vi "MainGlassCockpitWii.vi"() -> ()   [LabVIEW 2017]
uses:
  Sub_VIs/IMU_Functions/IMU_Data_Cluster.ctl
  Sub_VIs/Instruments/SlipIndicator.ctl
panel:
  out "Design":string
  out "Firmware Revision":string
  out "I2C Error Count":u16
  out "Cycle Time":u16
  out "Read Sensors":bool
  out "GPS-Fix":bool
  in  "EXIT":bool
  in  "ViewSelect":T1(tab)
  out "Boolesch 3":bool
  out "Boolesch 2":bool
  out "MultiWii Data Cluster OUT":T2 {"Altitude abs [m]" format="%.2f"; "Baro T [°C]" format="%.1f"; "Baro P [mbara]" format="%.1f"; "GPS_coord[LON]" format="%#_9f"; "GPS_coord[LAT]" format="%#_9f"; "Altitude [m]" format="%.2f"}
  out "No. of recorded Data":i32
  in  "Ident":bool
  in  "Status":bool
  in  "ACC_Calib.":bool
  in  "Mag_Calib.":bool
  in  "ReadSensorData":bool
  in  "RecordGPS-Data":bool
  in  "RecordFC-Data":bool
  out "COM ok":bool
  in  "COM Port":refnum<visa-resource-name>="COM7"
  in  "Difference Local/UTC [h]":i32=1
  out "GPS":string
  in  "GPS/Baro_Alt":bool
  in  "ScaleUnit(F=m; T=feet)":bool
  out "AltitudeIndicator":picture
  out "AltitudeDigital":dbl
  in  "GPS/Mag":bool
  in  "GPS/Baro_Vario":bool
  out "VerticalSpeedIndicator":picture
  out "VerticalSpeedDigital":dbl format="%.1f"
  out "HeadingDigital":dbl format="%.1f"
  out "TurnBankPlaneIndicator":picture caption="Neue Grafik"
  out "TurnBankStdRate":bool
  in  "ScaleUnit(F=km/h; T=knots)":bool
  out "SpeedIndicator":picture
  out "Local":string
  out "UTC":string
  out "ArtificialHorizon":picture
  out "SlipIndicator":T3 scale=-10.0..10.0
  out "Compass":picture
  # "Set the right COM port first before\nyou run the application !"
  # "on my laptop:\nCOM3-> SE v2.0\nCOM7-> AIOP v2.0"
  # "D - CF2811"
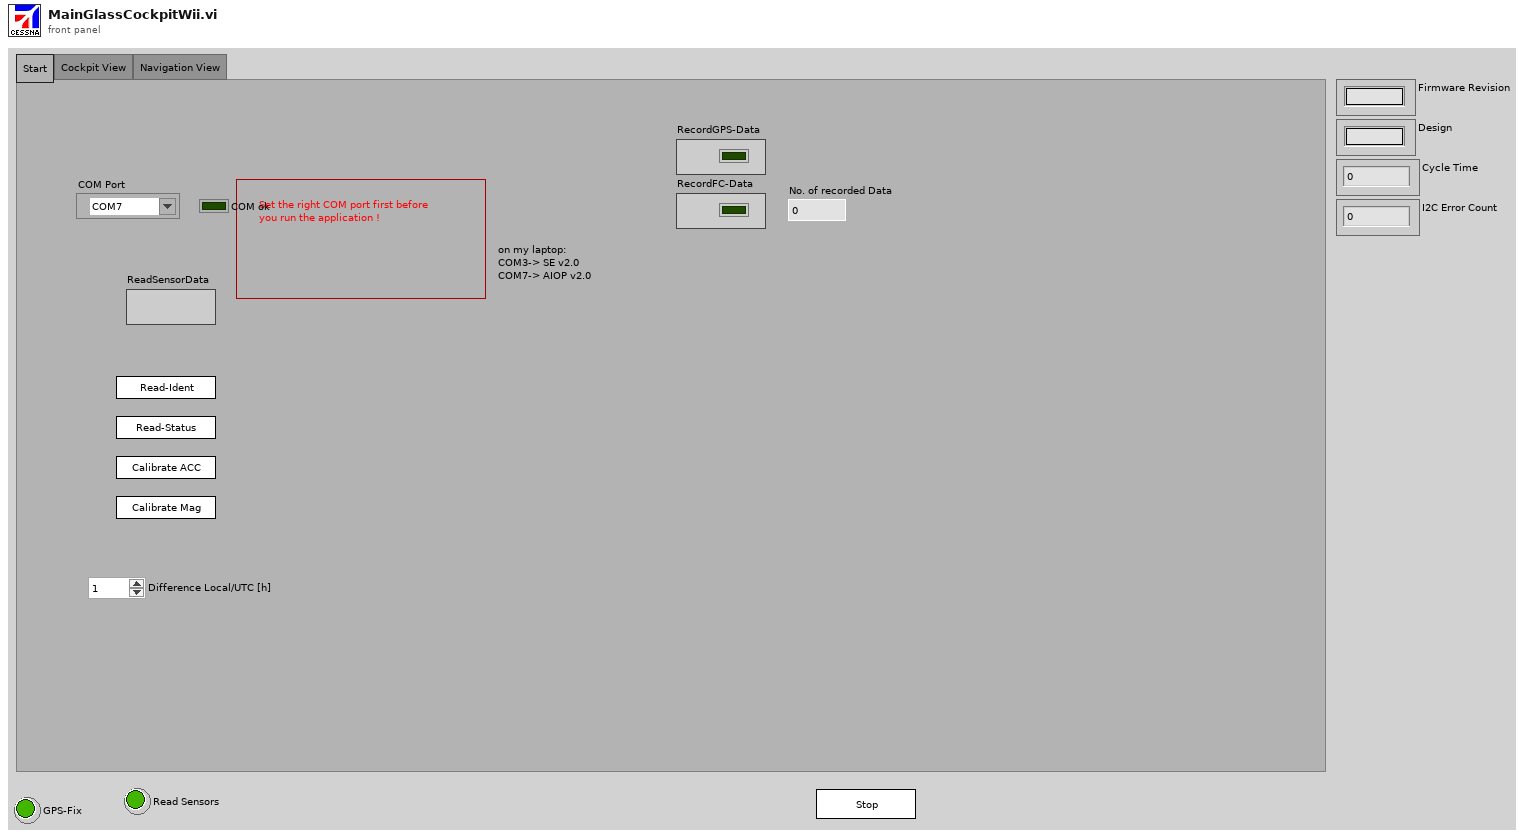
[diagram p1: front panel]
types:
  T1 = enum32{"Start", "Cockpit View", "Navigation View"}
  T2 = typedef "IMU_Data_Cluster.ctl" = cluster{"Firmware Revision":string, "Multitype Name":string, "Cycle Time":u16, "I²C Error Count":u16, "ACC present":bool, "Baro present":bool, "Mag Present":bool, "GPS present":bool, "Sonar present":bool, "Acc X axis (Roll)":dbl, "Acc Y axis (Pitch)":dbl, "Acc Z axis (Yaw)":dbl, "Gyro X axis (Roll)":dbl, "Gyro Y axis (Pitch)":dbl, "Gyro Z axis (Yaw)":dbl, "Mag X axis (Roll)":dbl, "Mag Y axis (Pitch)":dbl, "Mag Z axis (Yaw)":dbl, "X angle (Roll)":dbl, "Y angle (Pitch)":dbl, "Heading [°]":dbl, "Altitude [m]":dbl, "Vario":dbl, "GPS_Fix":u8, "GPS_NumSat":u8, "GPS_coord[LAT]":dbl, "GPS_coord[LON]":dbl, "GPS_Altitude":dbl, "GPS_Speed over Ground":dbl, "GPS_Ground Course":dbl, "Baro P [mbara]":dbl, "Baro T [°C]":dbl, "Altitude abs [m]":dbl}
  T3 = typedef "SlipIndicator.ctl" = dbl
  T4 = enum8{"Enabled", "Disabled", "Disabled and Grayed Out"}
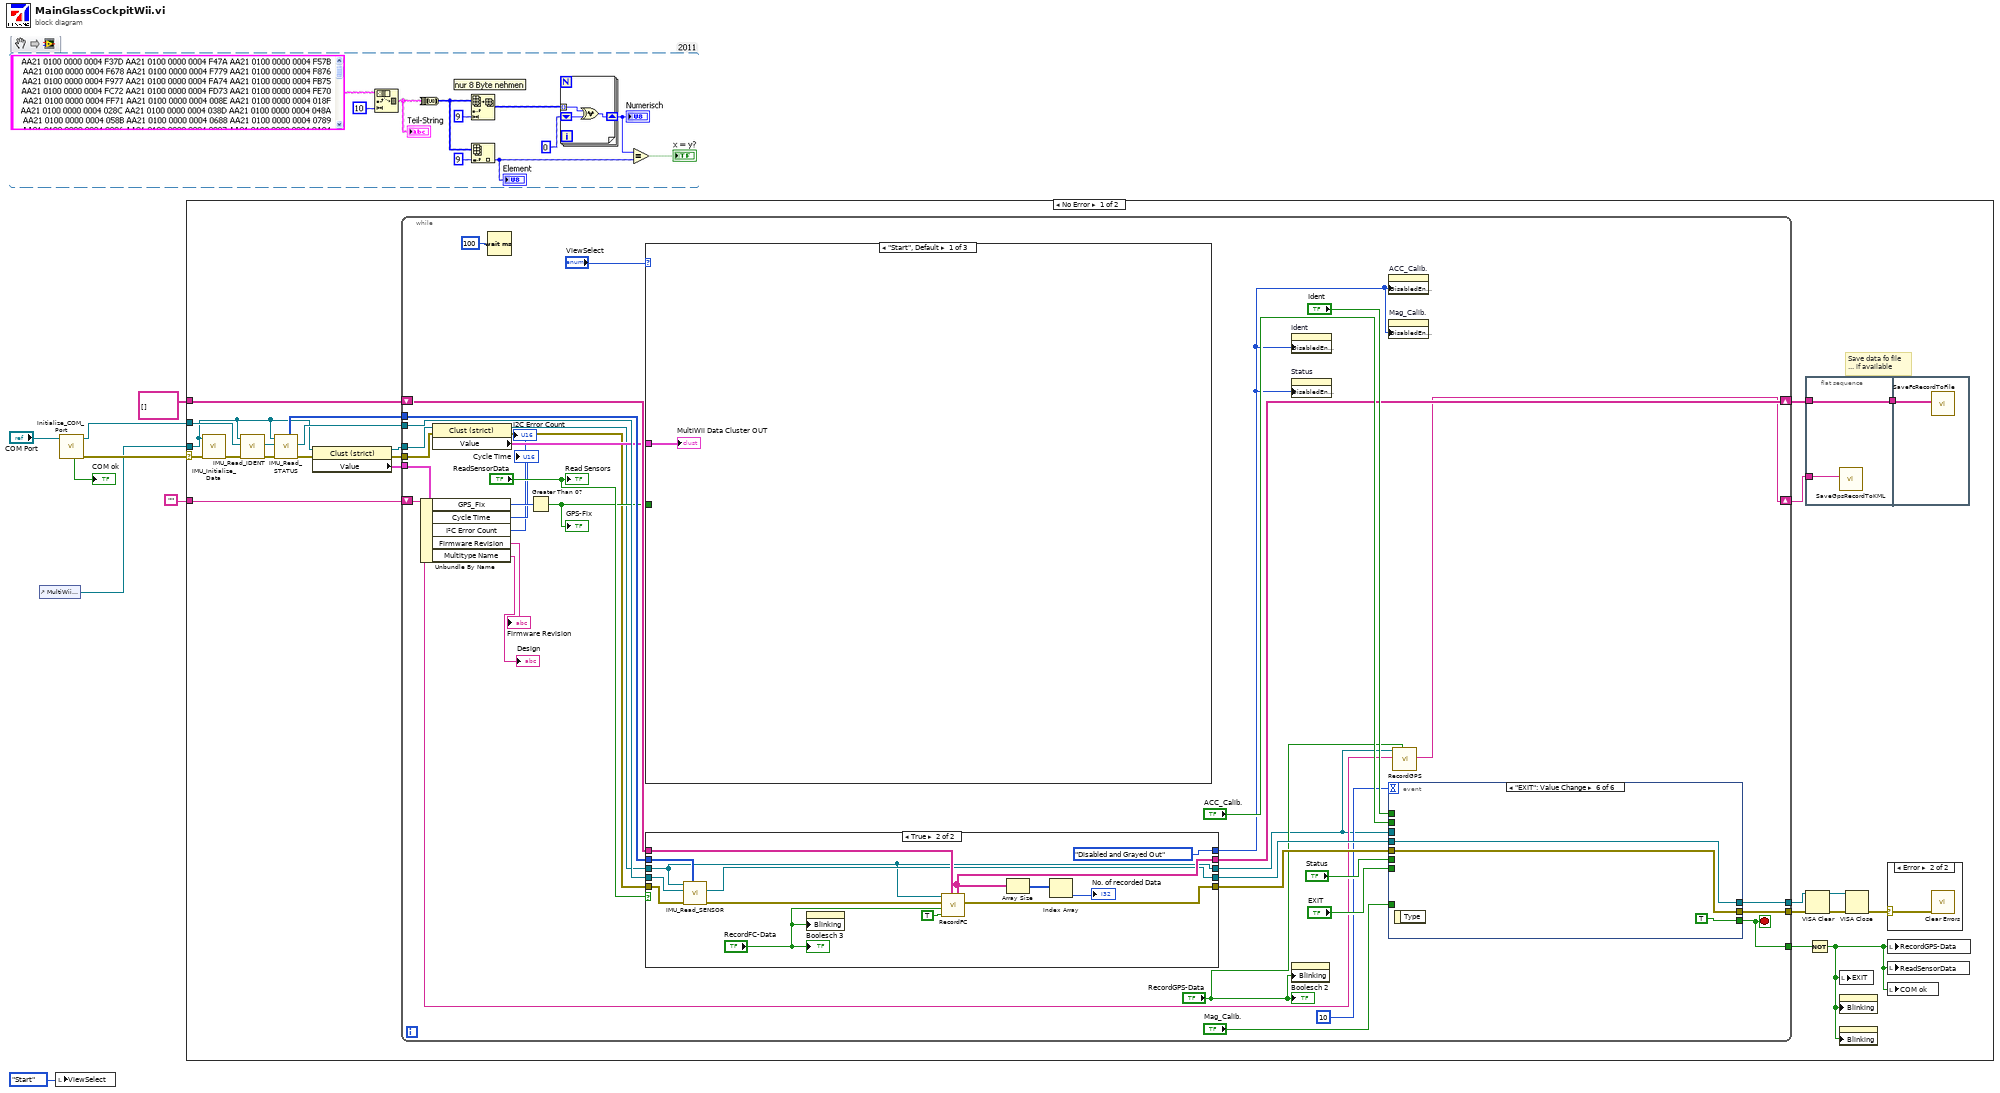
[diagram p0: block diagram]
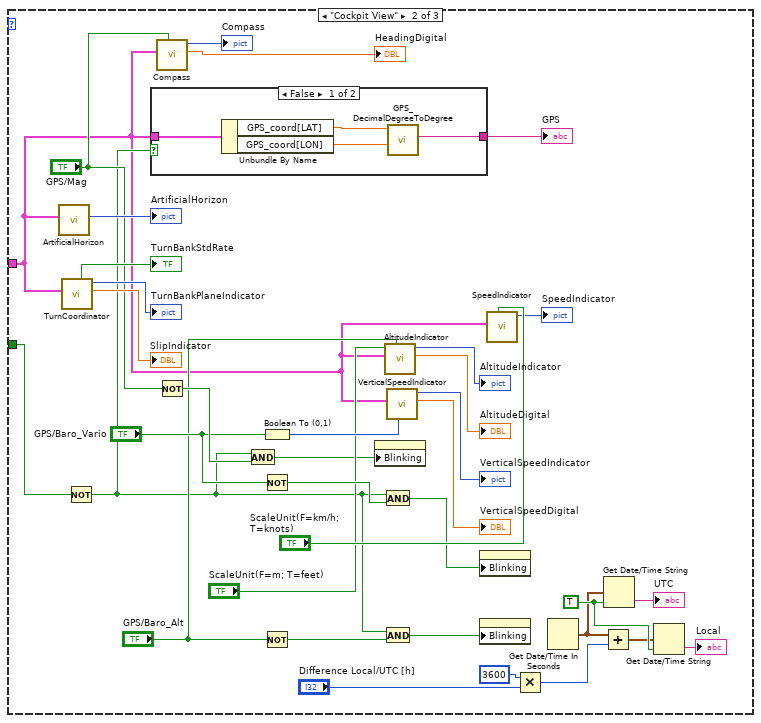
[diagram p3: hidden frame]
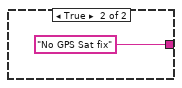
[diagram p4: hidden frame]
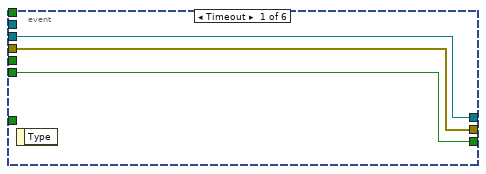
[diagram p6: hidden frame]
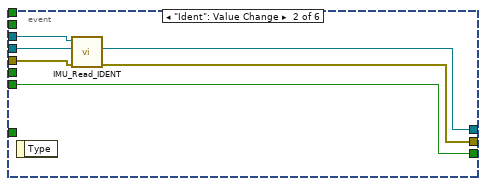
[diagram p7: hidden frame]
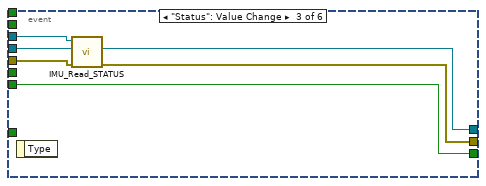
[diagram p8: hidden frame]
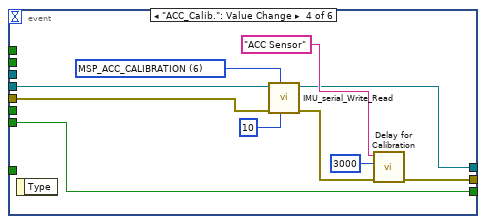
[diagram p9: hidden frame]
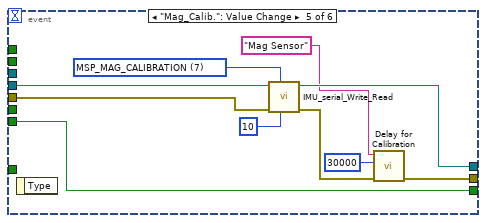
[diagram p10: hidden frame]
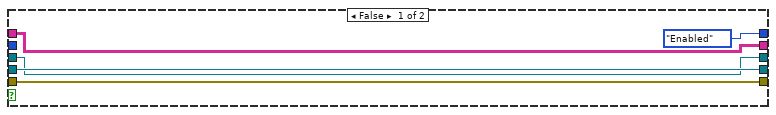
[diagram p11: hidden frame]
diagram:
  n1 = control-ref of="MultiWii Data Cluster OUT"() -> (w1:refnum<vi>)
  n2 = local write "ViewSelect"(T1."Start" ("ViewSelect")) -> ()
  n3 = call "Initialize_COM_Port.vi"("VISA resource name IN"="COM Port") -> ("error out 2"=w8:errorcluster, "VISA resource name OUT"=w7:refnum<visa-resource-name>, "COM ok"=→"COM ok":bool)  [unwired: 8 in]
  n4 = case shown="No Error" w8 {
    selector: w8 -> [w32 _]
    tunnel: w7 -> [w16 _]
    tunnel: "" -> [w22 _]
    tunnel: string[][] [] -> [w21 _]
    tunnel: w1 -> [w13 _]
    frame No Error {
      # "Save data fo file\n... if available"
      n5 = call "IMU_Initialize_Data.vi"("error in (no error)"=w32, "MultiWii Data Cluster"=w13) -> ("error out"=w31:errorcluster)  [unwired: 9 in]
      n6 = call "IMU_Read_IDENT.vi"("error in (no error)"=w31, "VISA resource name IN"=w16, "MultiWii Data Cluster 2"=w13) -> ("error out"=w30:errorcluster, "VISA resource name OUT"=w15:refnum<visa-resource-name>)  [unwired: 7 in]
      n7 = call "IMU_Read_STATUS.vi"("error in (no error)"=w30, "VISA resource name IN"=w15, "MultiWii Data Cluster 2"=w13) -> ("error out"=w12:errorcluster, "VISA resource name OUT"=w14:refnum<visa-resource-name>, "Sensors Present"=w23:u16[])  [unwired: 6 in]
      n8 = property class="Clust (strict)"(reference=w13, error in=w12) -> (reference out=w10:refnum<vi>, error out=w11:errorcluster, "Value"=w9:T2)
      n9 = while {
        tunnel: w14 -> [w71]
        tunnel: w11 -> [w42]
        tunnel: [w62] -> w25
        tunnel: [w64] -> w26
        tunnel: [w60] -> w29
        tunnel: w23 -> [w59]
        shift-right: [w52] -> w17
        shift-left: w22 -> [w53]
        shift-right: [w56] -> w18
        shift-left: w21 -> [w57]
        tunnel: w10 -> [w46]
        tunnel: w9 -> [w45]
        stop <- w60 stop-if-true
        n10 = Unbundle By Name(w45) -> ("GPS_Fix"=w49:u8, "Cycle Time"=→"Cycle Time":u16, "I²C Error Count"=→"I2C Error Count":u16, "Firmware Revision"=→"Firmware Revision":string, "Multitype Name"=→"Design":string)
        n11 = property class="Clust (strict)"(reference=w46, error in=w42) -> (reference out=w43:refnum<vi>, error out=w41:errorcluster, "Value"=w44:T2)
        n12 = Wait (ms)(milliseconds to wait=u32 100 ("Zu wartende ms")) -> ()  [unwired: 1 out]
        n13 = Greater Than 0?(x=w49) -> (x > 0?=w48:bool)
        "GPS-Fix" <- w48
        n14 = case shown="\"Start\", Default" "ViewSelect" {
          tunnel: w44 -> [w72 w74 _]
          tunnel: w48 -> [_ w76 _]
          frame "Start", Default {
            "MultiWii Data Cluster OUT" <- w72
          }
          frame "Cockpit View" {
            w102 = TRUE
            n15 = call "ArtificialHorizon.vi"("MultiWii Data Cluster"=w74) -> ("ArtificialHorizon"=→"ArtificialHorizon":picture)  [unwired: 9 in, 1 out]
            n16 = call "TurnCoordinator.vi"("MultiWii Data Cluster"=w74) -> ("SlipIndicator"=→"SlipIndicator":T3, "TurnBankPlaneIndicator"=→"TurnBankPlaneIndicator":picture, "TurnBankStdRate"=→"TurnBankStdRate":bool)  [unwired: 5 in, 3 out]
            n17 = Not(x=w76) -> (.not. x?=w75:bool)
            n18 = case shown="False" w75 {
              tunnel: [w111 "No GPS Sat fix"] -> w73
              tunnel: w74 -> [w110 _]
              frame False {
                n19 = Unbundle By Name(w110) -> ("GPS_coord[LAT]"=w109:dbl, "GPS_coord[LON]"=w108:dbl)
                n20 = call "GPS_DecimalDegreeToDegree.vi"("Lon(decimal degrees)"=w108, "Lat(decimal degrees)"=w109) -> ("GPS"=w111:string)  [unwired: 8 in, 1 out]
              }
              frame True {
              }
            }
            "GPS" <- w73
            n21 = call "Compass.vi"("GPS/Mag"="GPS/Mag", "MultiWii Data Cluster"=w74) -> ("Heading Digital"=→"HeadingDigital":dbl, "CompassGauge"=→"Compass":picture)  [unwired: 7 in, 1 out]
            n22 = Not(x="GPS/Mag") -> (.not. x?=w105:bool)
            n23 = And(x=w75, y=w105) -> (x .and. y?=w83:bool)
            n24 = Boolean To (0,1)(Boolean="GPS/Baro_Vario") -> (0, 1=w98:i16)
            n25 = Not(x="GPS/Baro_Vario") -> (.not. x?=w106:bool)
            n26 = Not(x="GPS/Baro_Alt") -> (.not. x?=w107:bool)
            n27 = property on="GPS/Mag" class="Bool (strict)"("Blinking"=w83) -> ()  [unwired: 2 in, 2 out]
            n28 = And(x=w75, y=w106) -> (x .and. y?=w79:bool)
            n29 = And(x=w75, y=w107) -> (x .and. y?=w77:bool)
            n30 = call "AltitudeIndicator.vi"("GPS/Baro_Alt"="GPS/Baro_Alt", "MultiWii Data Cluster"=w74, "ScaleUnit(F=m; T=feet)"="ScaleUnit(F=m; T=feet)") -> ("Altitude  (/10000)"=→"AltitudeDigital":dbl, "AltitudeIndicator"=→"AltitudeIndicator":picture)  [unwired: 4 in, 3 out]
            n31 = call "VerticalSpeedIndicator.vi"("SignalSource"=w98, "MultiWii Data Cluster"=w74) -> ("VerticalSpeedDigital"=→"VerticalSpeedDigital":dbl, "VerticalSpeedIndicator"=→"VerticalSpeedIndicator":picture)  [unwired: 7 in, 1 out]
            n32 = property on="GPS/Baro_Vario" class="Bool (strict)"("Blinking"=w79) -> ()  [unwired: 2 in, 2 out]
            n33 = property on="GPS/Baro_Alt" class="Bool (strict)"("Blinking"=w77) -> ()  [unwired: 2 in, 2 out]
            n34 = call "SpeedIndicator.vi"("ScaleUnit(F=km/h; T=knots)"="ScaleUnit(F=km/h; T=knots)", "MultiWii Data Cluster"=w74) -> ("SpeedIndicator"=→"SpeedIndicator":picture)  [unwired: 8 in, 1 out]
            n35 = Multiply(x=3600 ("number"), y="Difference Local/UTC [h]") -> (x*y=w103:i32)
            n36 = Get Date/Time In Seconds() -> (seconds since 1Jan1904=w100:timestamp)
            n37 = Add(x=w100, y=w103) -> (x+y=w101:timestamp)
            n38 = Get Date/Time String(seconds (now)=w100, want seconds? (F)=w102) -> (time string=→"UTC":string)  [unwired: 1 in, 1 out]
            n39 = Get Date/Time String(seconds (now)=w101, want seconds? (F)=w102) -> (time string=→"Local":string)  [unwired: 1 in, 1 out]
          }
          frame "Navigation View" {
          }
        }
        n40 = case shown="True" "ReadSensorData" {
          tunnel: w71 -> [w155 w158]
          tunnel: w41 -> [w154 w168]
          tunnel: [w155 w157] -> w65
          tunnel: [w154 w165] -> w63
          tunnel: [T4."Enabled" ("Deaktiviert") T4."Disabled and Grayed Out" ("Deaktiviert")] -> w54
          tunnel: w59 -> [_ w167]
          tunnel: w57 -> [w152 w163]
          tunnel: [w152 w160] -> w56
          tunnel: w43 -> [w151 w156]
          tunnel: [w151 w156] -> w47
          frame False {
          }
          frame True {
            n41 = call "IMU_Read_SENSOR.vi"("Sensors Present"=w167, "error in (no error)"=w168, "VISA resource name IN"=w158, "MultiWii Data Cluster 2"=w156) -> ("error out"=w166:errorcluster, "VISA resource name OUT"=w157:refnum<visa-resource-name>)  [unwired: 6 in]
            n42 = property on="Boolesch 3" class="Bool (strict)"("Blinking"="RecordFC-Data") -> ()  [unwired: 2 in, 2 out]
            n43 = call "RecordFC.vi"("FC-Data"=w163, "Latching"=TRUE, "RecordFCdata"="RecordFC-Data", "error in (no error)"=w166, "MultiWii Data Cluster 2"=w156) -> ("error out"=w165:errorcluster, "FC-Data OUT"=w160:string[][])  [unwired: 5 in]
            n44 = Array Size(array=w160) -> (size(s)=w161:i32[])
            n45 = Index Array(array=w161) -> (element=→"No. of recorded Data":i32)  [unwired: 1 in]
            "Boolesch 3" <- "RecordFC-Data"
          }
        }
        n46 = property on="Ident" class="Bool"("DisabledEnum"=w54) -> ()  [unwired: 2 in, 2 out]
        n47 = property on="Status" class="Bool"("DisabledEnum"=w54) -> ()  [unwired: 2 in, 2 out]
        n48 = property on="Boolesch 2" class="Bool (strict)"("Blinking"="RecordGPS-Data") -> ()  [unwired: 2 in, 2 out]
        n49 = property on="ACC_Calib." class="Bool"("DisabledEnum"=w54) -> ()  [unwired: 2 in, 2 out]
        n50 = property on="Mag_Calib." class="Bool"("DisabledEnum"=w54) -> ()  [unwired: 2 in, 2 out]
        n51 = event shown="[5] \"EXIT\": Value Change" {
          selector: _ -> [_ _ _ _ _ _]
          dyn-events: _ -> [_ _ _ _ _ _]
          timeout: 10 -> [_ _ _ _ _ _]
          tunnel: "EXIT" -> [w115 w121 w127 w137 w147 _]
          tunnel: "Mag_Calib." -> [_ _ _ _ _ _]
          tunnel: "ACC_Calib." -> [_ _ _ _ _ _]
          tunnel: "Status" -> [_ _ _ _ _ _]
          tunnel: "Ident" -> [_ _ _ _ _ _]
          tunnel: [w115 w121 w127 w137 w147 TRUE ("EXIT")] -> w60
          tunnel: w65 -> [w114 w117 w123 w136 w146 w150]
          tunnel: [w114 w118 w122 w129 w140 w150] -> w64
          tunnel: w63 -> [w113 w120 w126 w135 w145 w149]
          tunnel: [w113 w119 w125 w130 w142 w149] -> w62
          tunnel: w47 -> [_ w116 w124 _ _ _]
          event Timeout {
            n52 = event-data() -> ()  [unwired: 1 in, 1 out]
          }
          event "Ident": Value Change {
            n53 = event-data() -> ()  [unwired: 1 in, 1 out]
            n54 = call "IMU_Read_IDENT.vi"("error in (no error)"=w120, "VISA resource name IN"=w117, "MultiWii Data Cluster 2"=w116) -> ("error out"=w119:errorcluster, "VISA resource name OUT"=w118:refnum<visa-resource-name>)  [unwired: 7 in]
          }
          event "Status": Value Change {
            n55 = event-data() -> ()  [unwired: 1 in, 1 out]
            n56 = call "IMU_Read_STATUS.vi"("error in (no error)"=w126, "VISA resource name IN"=w123, "MultiWii Data Cluster 2"=w124) -> ("error out"=w125:errorcluster, "VISA resource name OUT"=w122:refnum<visa-resource-name>)  [unwired: 6 in, 1 out]
          }
          event "ACC_Calib.": Value Change {
            w134 = u16 6 items=["MSP_IDENT", "MSP_STATUS", "MSP_RAW_IMU", "MSP_RAW_GPS", "MSP_ATTITUDE", "MSP_ALTITUDE", "MSP_ACC_CALIBRATION", "MSP_MAG_CALIBRATION"] ("Command Selection")
            n57 = event-data() -> ()  [unwired: 1 in, 1 out]
            n58 = call "IMU_serial_Write_Read.vi"("Delay (ms)"=u32 10, "Command Selection"=w134, "error in (no error)"=w135, "VISA resource name IN"=w136) -> ("error IO"=w131:errorcluster, "VISA resource name OUT"=w129:refnum<visa-resource-name>)  [unwired: 5 in, 1 out]
            n59 = call "Delay for Calibration.vi"("Error In"=w131, "Delay (ms)"=3000, "Frame Name"="ACC Sensor") -> ("Error Out"=w130:errorcluster)  [unwired: 8 in]
          }
          event "Mag_Calib.": Value Change {
            w144 = u16 7 items=["MSP_IDENT", "MSP_STATUS", "MSP_RAW_IMU", "MSP_RAW_GPS", "MSP_ATTITUDE", "MSP_ALTITUDE", "MSP_ACC_CALIBRATION", "MSP_MAG_CALIBRATION"] ("Command Selection")
            n60 = event-data() -> ()  [unwired: 1 in, 1 out]
            n61 = call "IMU_serial_Write_Read.vi"("Delay (ms)"=u32 10, "Command Selection"=w144, "error in (no error)"=w145, "VISA resource name IN"=w146) -> ("error IO"=w141:errorcluster, "VISA resource name OUT"=w140:refnum<visa-resource-name>)  [unwired: 5 in, 1 out]
            n62 = call "Delay for Calibration.vi"("Error In"=w141, "Delay (ms)"=30000, "Frame Name"="Mag Sensor") -> ("Error Out"=w142:errorcluster)  [unwired: 8 in]
          }
          event "EXIT": Value Change {
            n63 = event-data() -> ()  [unwired: 1 in, 1 out]
          }
        }
        n64 = call "RecordGPS.vi"("RecordGPS-Data"="RecordGPS-Data", "GPS_DataLog"=w53, "MultiWii Data Cluster 2"=w47) -> ("GPS_DataLogOut"=w52:string)  [unwired: 8 in]
        "Read Sensors" <- "ReadSensorData"
        "Boolesch 2" <- "RecordGPS-Data"
      }
      n65 = flat-sequence {
        tunnel: w17 -> [w34]
        tunnel: [w33] -> w20
        tunnel: w18 -> [w33]
        tunnel: w20 -> [w35]
        frame #0 {
          n66 = call "SaveGpsRecordToKML.vi"("GPS_LogData"=w34) -> ()  [unwired: 10 in, 1 out]
        }
        frame #1 {
          n67 = call "SaveFcRecordToFile.vi"("FC-Data"=w35) -> ()  [unwired: 10 in, 1 out]
        }
      }
      n68 = VISA Clear(VISA resource name=w26, error in (no error)=w25) -> (VISA resource name out=w28:refnum<visa-resource-name>, error out=w27:errorcluster)
      n69 = Not(x=w29) -> (.not. x?=w19:bool)
      n70 = local write "EXIT"(w19) -> ()
      n71 = property on="Boolesch 3" class="Bool (strict)"("Blinking"=w19) -> ()  [unwired: 2 in, 2 out]
      n72 = property on="Boolesch 2" class="Bool (strict)"("Blinking"=w19) -> ()  [unwired: 2 in, 2 out]
      n73 = VISA Close(VISA resource name=w28, error in (no error)=w27) -> (error out=w24:errorcluster)
      n74 = case shown="Error" w24 {
        selector: w24 -> [_ w36]
        frame No Error {
        }
        frame Error {
          n75 = call <vilib>:"Clear Errors.vi"("error in (no error)"=w36) -> ()  [unwired: 5 in, 2 out]
        }
      }
      n76 = local write "RecordGPS-Data"(w19) -> ()
      n77 = local write "ReadSensorData"(w19) -> ()
      n78 = local write "COM ok"(w19) -> ()
    }
    frame Error {
    }
  }
